vi "Config Lines to array.vi"(7 "section":string, 8 "error in (no error)":errorcluster, 10 "Key Name":string, 11 "Refnum in":T1) -> (0 "error out":errorcluster, 2 "Array":string[](array[string]), 3 "Refnum out":T1)   [LabVIEW 2015, in "SLSC Switch.lvclass"]
uses:
  SLSC Switch.lvclass
  <vilib>/Utility/config.llb/Config Data RefNum.ctl
  <vilib>/Utility/config.llb/Read Key (String).vi
  <vilib>/Utility/config.llb/NI_LVConfig.lvlib
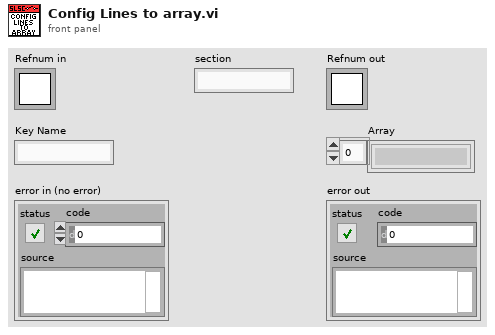
[diagram p1: front panel]
types:
  T1 = typedef "NI_LVConfig.lvlib/Config Data RefNum.ctl" = refnum<k1>
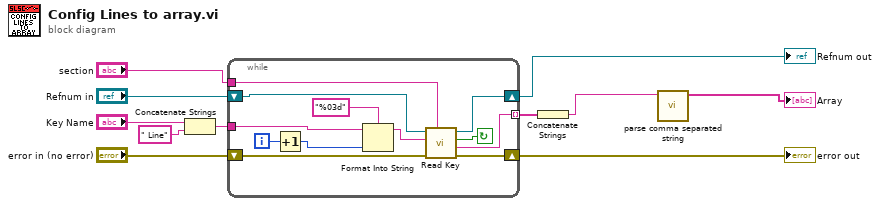
[diagram p0: block diagram]
diagram:
  n1 = Concatenate Strings("Key Name", " Line" ("string")) -> (w11:string)
  n2 = while {
    tunnel: [w19] -> w3 mode=indexing
    shift-right: [w15] -> w4
    shift-left: "Refnum in" -> [w22]
    shift-right: [w14] -> w7
    shift-left: "error in (no error)" -> [w23]
    tunnel: "section" -> [w13]
    tunnel: w11 -> [w12]
    i -> [w16]
    stop <- w18 continue-if-true
    n3 = Increment(x=w16) -> (x+1=w17:i32)
    n4 = Format Into String(format string="%03d", initial string=w12, w17) -> (resulting string=w20:string)  [unwired: 1 in, 1 out]
    n5 = call-poly <vilib>:"Read Key.vi"("section"=w13, "error in (no error)"=w23, "key"=w20, "refnum"=w22) -> ("error out"=w14:errorcluster, "value"=w19:string, "found?"=w18:bool, "refnum out"=w15:T1)  [unwired: 4 in]
  }
  "error out" <- w7
  "Refnum out" <- w4
  n6 = Concatenate Strings(w3) -> (w5:string)
  n7 = call "parse comma separated string.vi"("String"=w5) -> ("Array"=→"Array":string[])  [unwired: 10 in]
